vi "Linear to dB (array).vi"(1 "linear":dbl[](array[numeric])) -> (0 "dB":dbl[](array[numeric]))   [LabVIEW 2020]
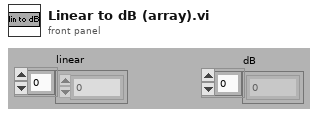
[diagram p1: front panel]
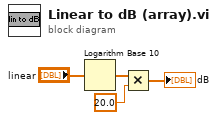
[diagram p0: block diagram]
diagram:
  n1 = Logarithm Base 10(1:"linear") -> (0:w3:dbl[])
  n2 = Multiply(x=w3, y=20.0) -> (x*y=→"dB":dbl[])
